vi "Current_Training_UI_3.10.22.vi"() -> ()   [LabVIEW 2021]
panel:
  out "Console out":string
  out "intro":picture
  out "view":picture
  out "training 2":picture
  out "sent string":string
  out "training":u16[](array[numeric])
  out "Motor Value":i32
  in  "Quit":bool
  out "Training String":string
  out "Tab Control":enum32{"Welcome", "View", "Train"}(tab)
  in  "Ready":bool
  out "Motor Position View":u8(knob) scale=0.0..4.0
  in  "TRAIN":bool
  out "Light Intensity % View":dbl(slide) scale=0.0..100.0
  out "?":u32(colorbox)
  in  "Done":bool
  in  "Motor Position":u8(knob) scale=0.0..4.0
  out "Light Intensity %":dbl(slide) scale=0.0..100.0
  in  "Training Data":bool
  in  "Upload":bool
  out "Light Intensity 2":u32(colorbox)
  out "table":picture
  in  "Done 2":bool
  out "concatenated string":string
  out "read buffer":string
  out "Motor":string
  out "Sensor":string
  out "Type":string
  out "Name":string
  out "read terminal buffer - view":string
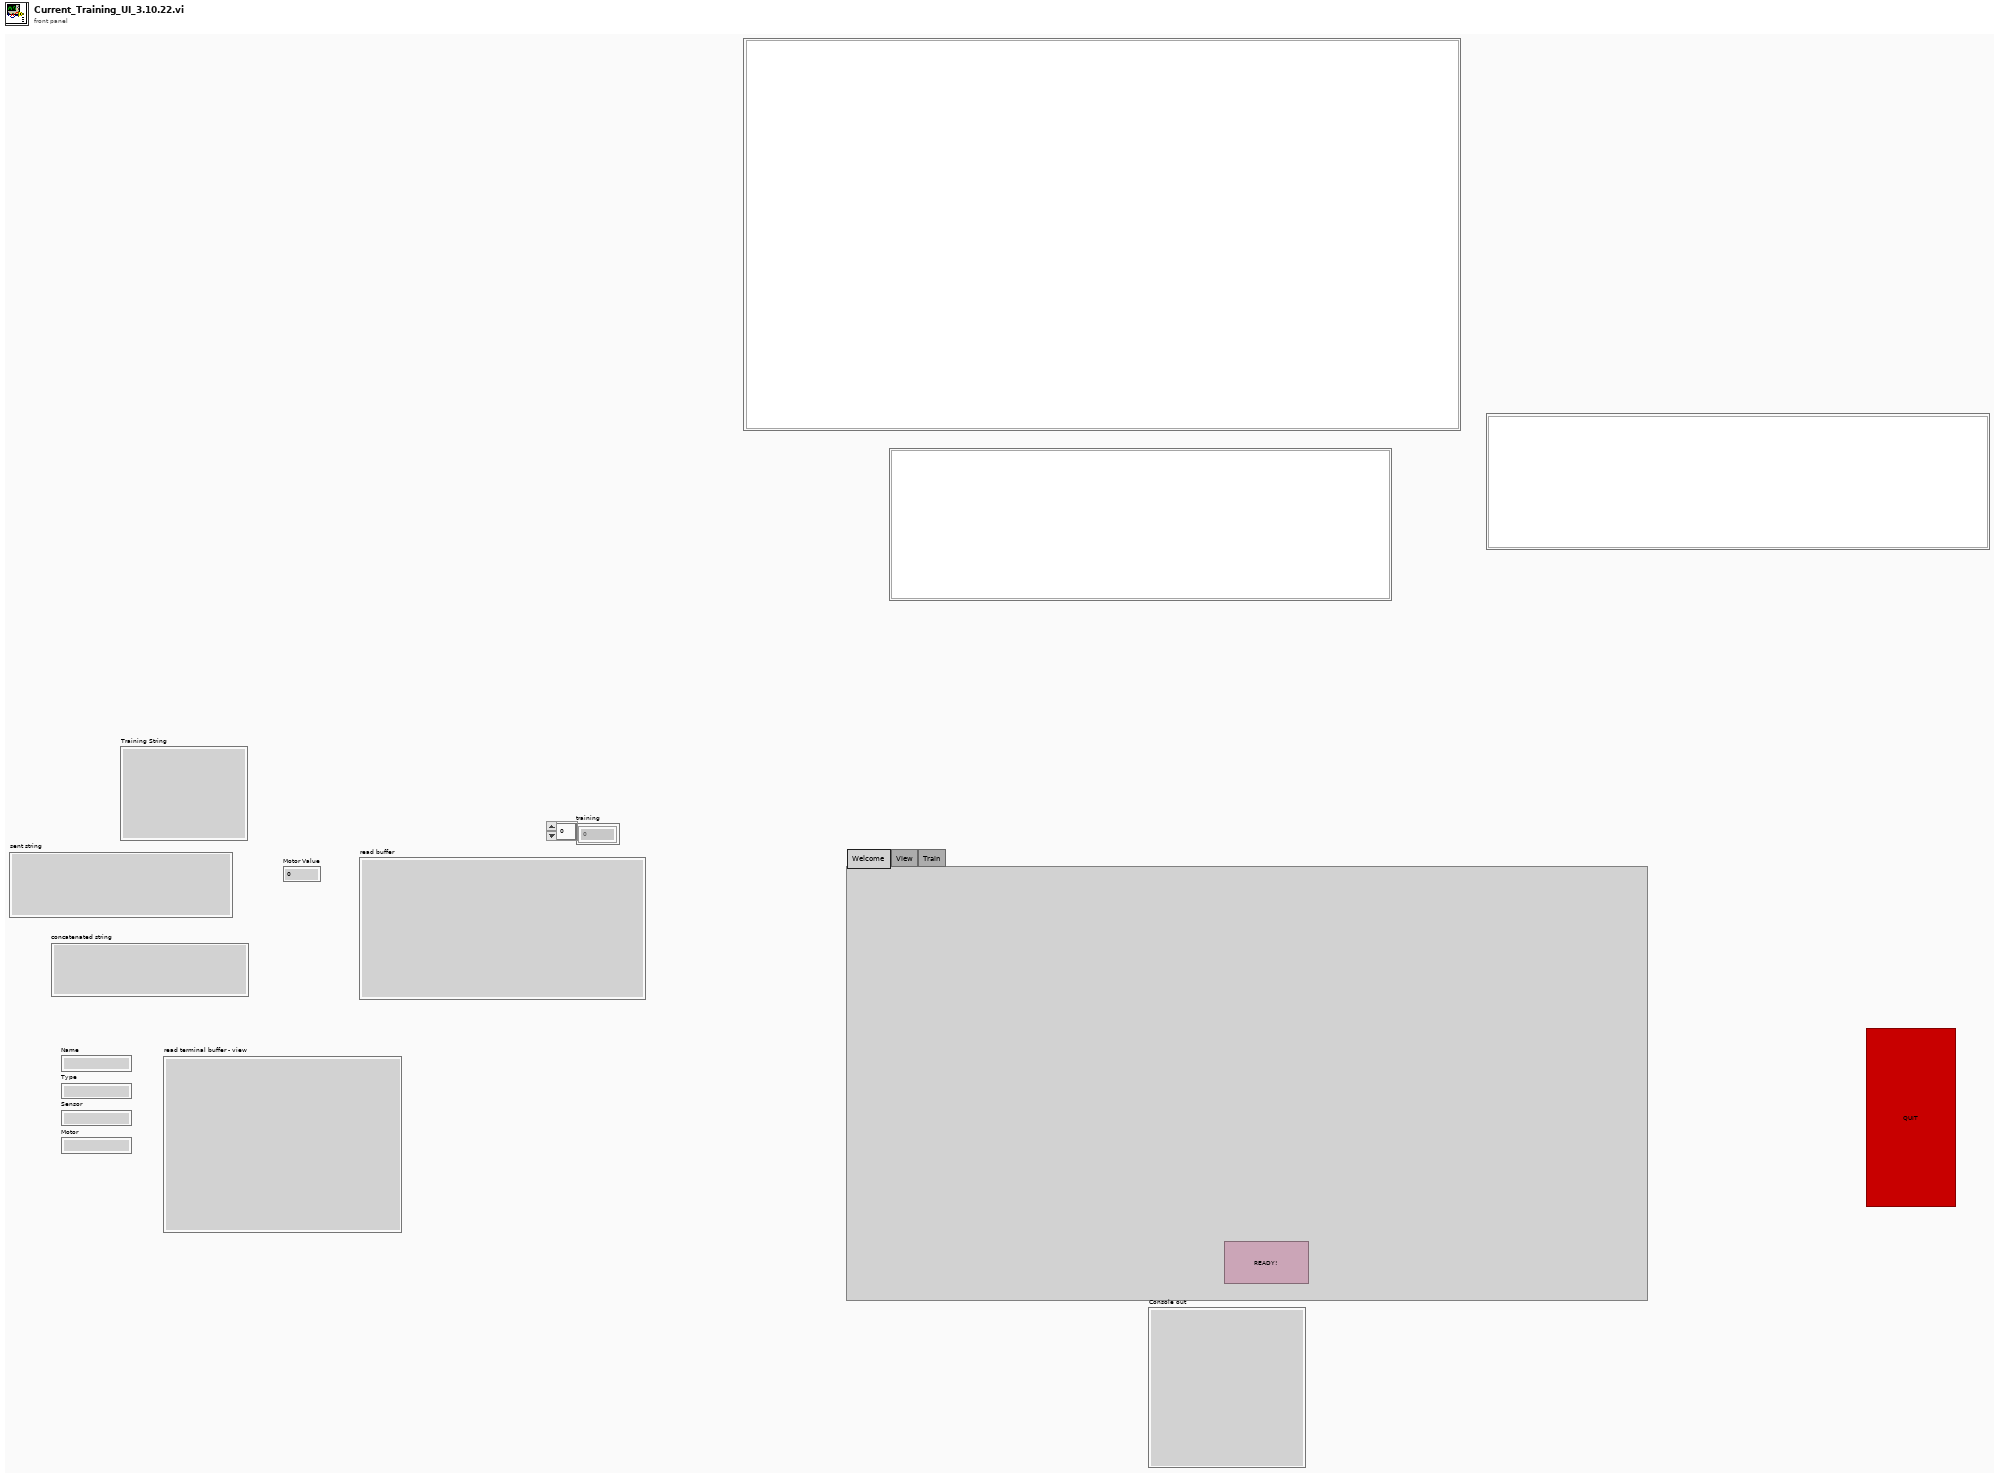
[diagram p1: front panel]
types:
  T1 = typedef "PythonCtrl.ctl" = cluster{"session":refnum<k35>, "PyPath":path, "Processor":enum16{"SPIKE", "Pi", "Pi_ssh"}}
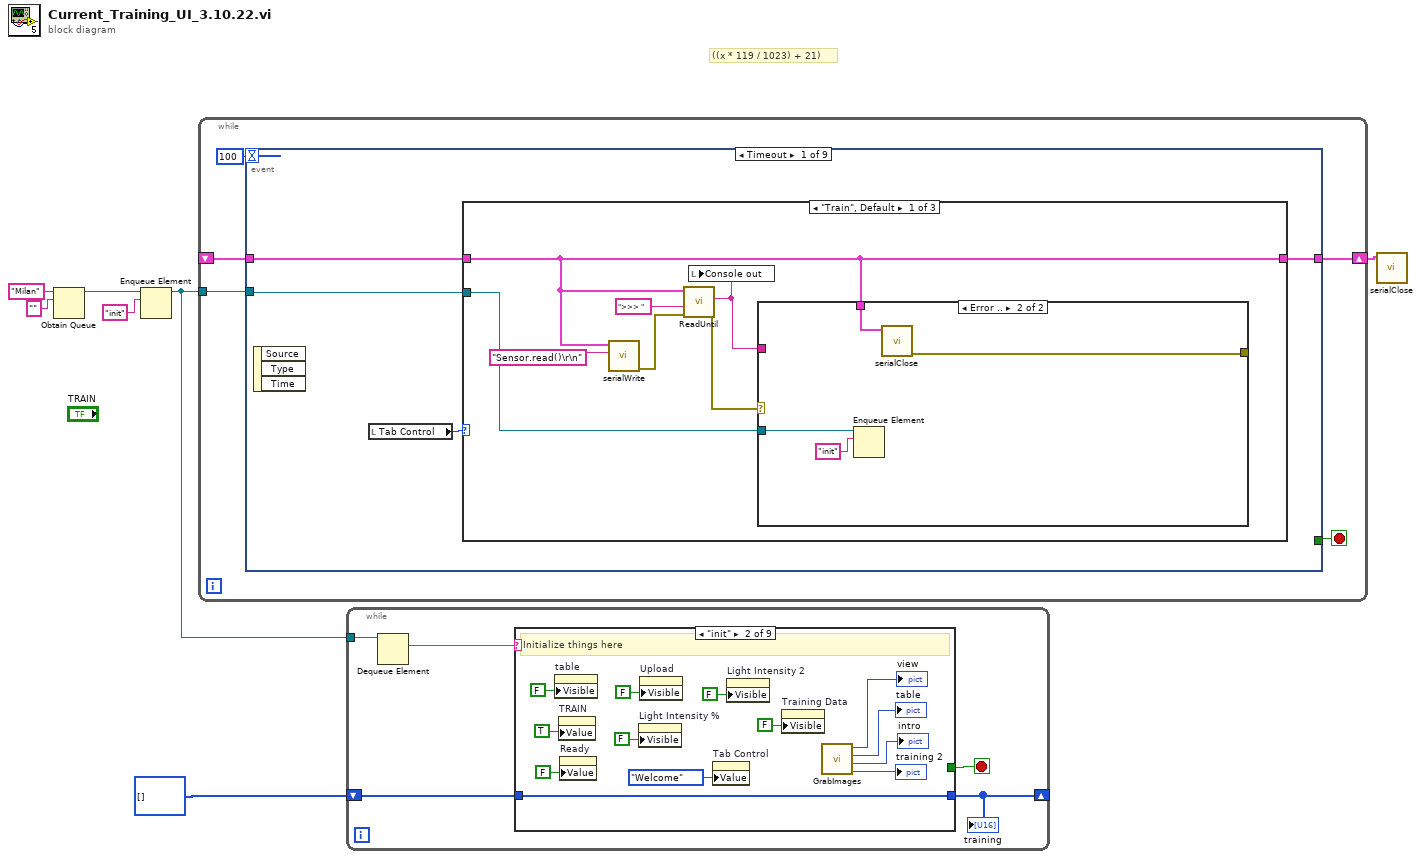
[diagram p0: block diagram]
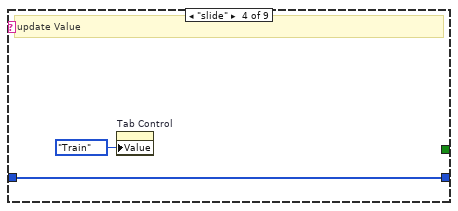
[diagram p4: hidden frame]
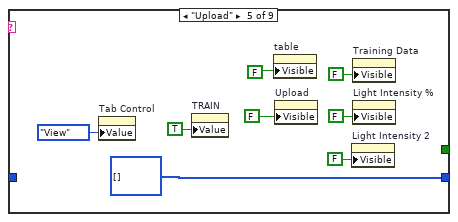
[diagram p5: hidden frame]
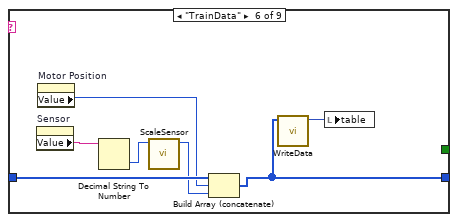
[diagram p6: hidden frame]
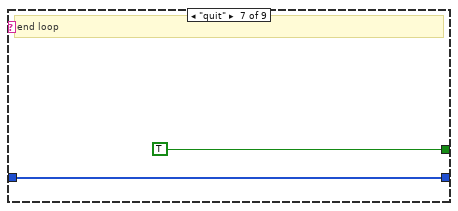
[diagram p7: hidden frame]
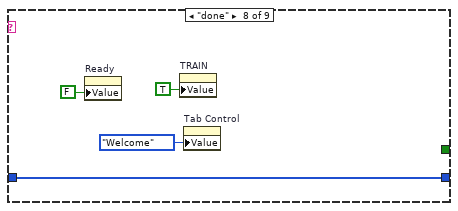
[diagram p8: hidden frame]
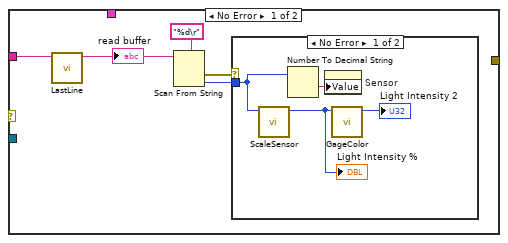
[diagram p10: hidden frame]
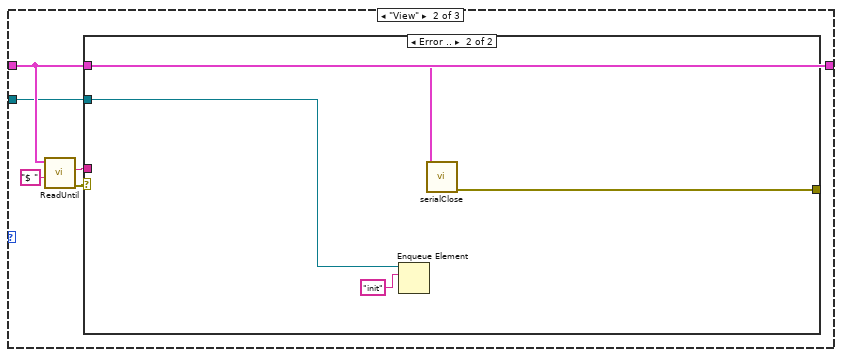
[diagram p12: hidden frame]
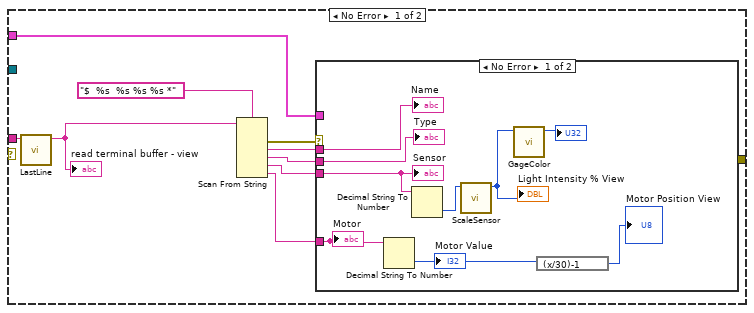
[diagram p13: hidden frame]
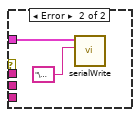
[diagram p14: hidden frame]
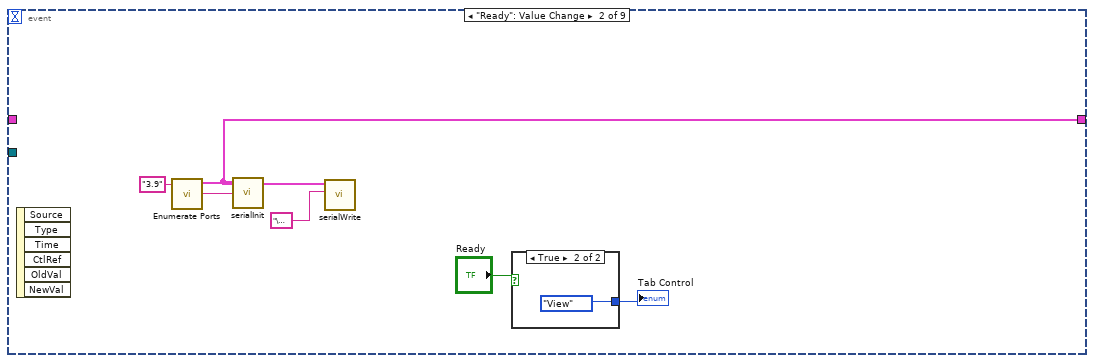
[diagram p16: hidden frame]
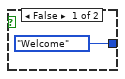
[diagram p17: hidden frame]
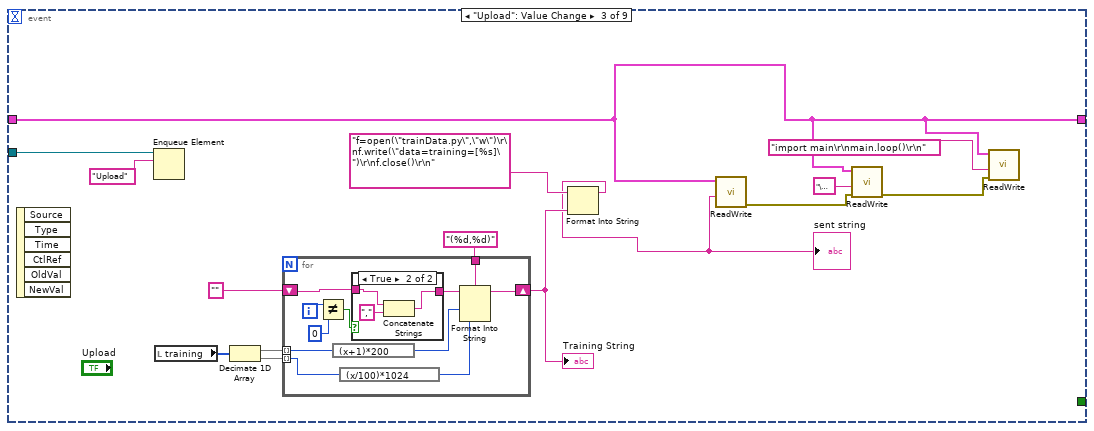
[diagram p18: hidden frame]
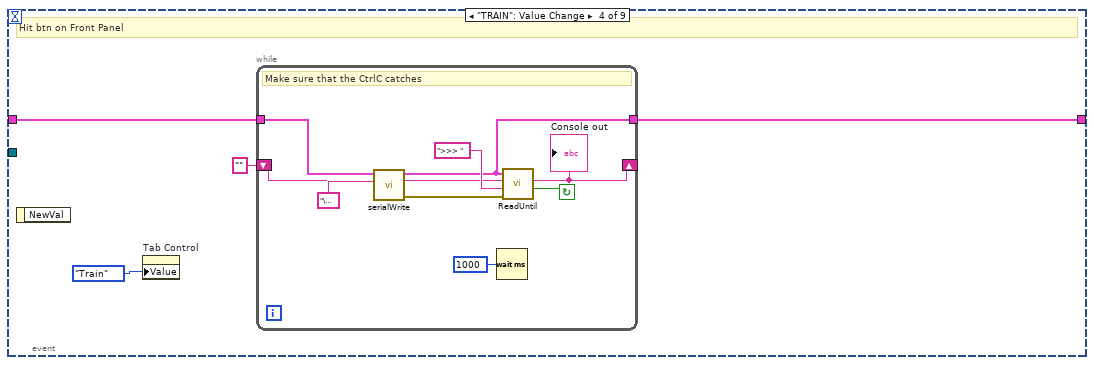
[diagram p20: hidden frame]
diagram:
  # "((x * 119 / 1023) + 21)"
  n1 = Obtain Queue(name (unnamed)="Milan", element data type="") -> (queue out=w7:refnum<queue>)  [unwired: 3 in, 2 out]
  n2 = Enqueue Element(queue=w7, element="init") -> (queue out=w3:refnum<queue>)  [unwired: 2 in, 2 out]
  n3 = while {
    tunnel: w3 -> [w12]
    shift-right: [w9] -> w2
    shift-left: _ -> [w10]
    stop <- w11 stop-if-true
    n4 = event shown="[0] Timeout" {
      selector: _ -> [_ _ _ _ _ _ _ _ _]
      dyn-events: _ -> [_ _ _ _ _ _ _ _ _]
      timeout: 100 -> [_ _ _ _ _ _ _ _ _]
      tunnel: w12 -> [w13 _ w89 _ w120 w130 w134 w138 w143]
      tunnel: [_ _ _ _ _ _ w133 TRUE ("Discard?") _] -> w11
      tunnel: w10 -> [w15 _ w75 w107 w119 w129 w132 w136 w140]
      tunnel: [w16 w67 w75 w106 w119 w129 w132 w136 w140] -> w9
      event Timeout {
        n5 = event-data() -> ()  [unwired: 1 in, 3 out]
        n6 = local read "Tab Control"() -> (w14:enum32{"Welcome", "View", "Train"})
        n7 = case shown="\"Train\", Default" w14 {
          tunnel: w15 -> [w18 w41 w66]
          tunnel: [w18 w41 w66] -> w16
          tunnel: w13 -> [w17 w37 _]
          frame "Train", Default {
            n8 = call "serialWrite.vi"("text"="Sensor.read()\r\n" ("write buffer"), "Python"=w18) -> ("error out"=w21:errorcluster)  [unwired: 8 in, 1 out]
            n9 = call "ReadUntil.vi"("error in (no error)"=w21, "EOL"=">>> ", "Python"=w18) -> ("error out"=w19:errorcluster, "Console out"=w20:string)  [unwired: 6 in, 1 out]
            n10 = local write "Console out"(w20) -> ()
            n11 = case shown="Error .." w19 {
              tunnel: w20 -> [w24 _]
              tunnel: w18 -> [_ w35]
              tunnel: w17 -> [_ w34]
              tunnel: [_ w33] -> _
              frame No Error {
                n12 = call "LastLine.vi"("Reply"=w24) -> ("String"=w25:string)  [unwired: 10 in]
                "read buffer" <- w25
                n13 = Scan From String(format string="%d\r", input string=w25) -> (error out=w28:errorcluster, output 1=w27:i32)  [unwired: 3 in, 2 out]
                n14 = case shown="No Error" w28 {
                  tunnel: w27 -> [w30 _]
                  frame No Error {
                    n15 = call "ScaleSensor.vi"("value"=w30) -> ("scaled value"=w29:u16)  [unwired: 10 in]
                    "Light Intensity %" <- w29
                    n16 = Number To Decimal String(number=w30) -> (decimal integer string=w32:string)  [unwired: 1 in]
                    n17 = property on="Sensor" class="Str"("Value"=w32) -> ()  [unwired: 2 in, 2 out]
                    n18 = call "GageColor.vi"("value"=w29) -> ("Color Box"=→"Light Intensity 2":u32)  [unwired: 10 in]
                  }
                  frame Error {
                  }
                }
              }
              frame Error {
                n19 = Enqueue Element(queue=w34, element="init") -> ()  [unwired: 2 in, 3 out]
                n20 = call "serialClose.vi"("Python in"=w35) -> ("error out"=w33:errorcluster)  [unwired: 10 in]
              }
            }
          }
          frame "View" {
            n21 = call "ReadUntil.vi"("EOL"="$ ", "Python"=w41) -> ("error out"=w39:errorcluster, "Console out"=w40:string)  [unwired: 7 in, 1 out]
            n22 = case shown="Error .." w39 {
              tunnel: w40 -> [w44 _]
              tunnel: w41 -> [w42 w64]
              tunnel: w37 -> [_ w63]
              tunnel: [_ w62] -> _
              frame No Error {
                n23 = call "LastLine.vi"("Reply"=w44) -> ("String"=w43:string)  [unwired: 10 in]
                "read terminal buffer - view" <- w43
                n24 = Scan From String(format string="$  %s  %s %s %s *", input string=w43) -> (error out=w50:errorcluster, output 1=w46:string, output 2=w47:string, output 3=w48:string, output 4=w49:string)  [unwired: 6 in, 2 out]
                n25 = case shown="No Error" w50 {
                  tunnel: w46 -> [w59 _]
                  tunnel: w47 -> [w58 _]
                  tunnel: w48 -> [w57 _]
                  tunnel: w49 -> [w54 _]
                  tunnel: w42 -> [_ w61]
                  frame No Error {
                    n26 = Decimal String To Number(string=w54) -> (number=w52:i32)  [unwired: 2 in, 1 out]
                    "Motor Value" <- w52
                    n27 = Decimal String To Number(string=w57) -> (number=w56:i32)  [unwired: 2 in, 1 out]
                    n28 = call "ScaleSensor.vi"("value"=w56) -> ("scaled value"=w53:u16)  [unwired: 10 in]
                    "Light Intensity % View" <- w53
                    n29 = call "GageColor.vi"("value"=w53) -> ("Color Box"=→"?":u32)  [unwired: 10 in]
                    n30 = expression code="(x/30)-1"(w52) -> (→"Motor Position View":i32)
                    "Name" <- w59
                    "Type" <- w58
                    "Sensor" <- w57
                    "Motor" <- w54
                  }
                  frame Error {
                    n31 = call "serialWrite.vi"("text"="\u0003", "Python"=w61) -> ()  [unwired: 8 in, 2 out]
                  }
                }
              }
              frame Error {
                n32 = Enqueue Element(queue=w63, element="init") -> ()  [unwired: 2 in, 3 out]
                n33 = call "serialClose.vi"("Python in"=w64) -> ("error out"=w62:errorcluster)  [unwired: 10 in]
              }
            }
          }
          frame "Welcome" {
          }
        }
      }
      event "Ready": Value Change {
        n34 = event-data() -> ()  [unwired: 1 in, 6 out]
        n35 = call "Enumerate Ports.vi"("Python version"="3.9") -> ("guess"=w70:string, "Python"=w67:T1)  [unwired: 6 in, 3 out]
        n36 = call "serialInit.vi"("Port"=w70, "Python"=w67) -> ()  [unwired: 8 in, 2 out]
        n37 = call "serialWrite.vi"("text"="\u0004" ("write buffer"), "Python"=w67) -> ()  [unwired: 8 in, 2 out]
        n38 = case shown="True" "Ready" {
          tunnel: [enum32{"Welcome", "View", "Train"}."Welcome" ("Tab Control") enum32{"Welcome", "View", "Train"}."View" ("Tab Control")] -> w71
          frame False {
          }
          frame True {
          }
        }
        "Tab Control" <- w71
      }
      event "Upload": Value Change {
        n39 = event-data() -> ()  [unwired: 1 in, 6 out]
        n40 = Enqueue Element(queue=w89, element="Upload") -> ()  [unwired: 2 in, 3 out]
        n41 = local read "training"() -> (w87:u16[])
        n42 = Decimate 1D Array(w87) -> (w85:u16[], w84:u16[])
        n43 = for {
          tunnel: "(%d,%d)" ("format string") -> [w100]
          tunnel: w85 -> [w93] mode=indexing
          tunnel: w84 -> [w91] mode=indexing
          shift-right: [w99] -> w82
          shift-left: "" -> [w98]
          i -> [w95]
          n44 = Not Equal?(x=w95, y=0) -> (x != y?=w96:bool)
          n45 = expression code="(x+1)*200"(w93) -> (w92:u16)
          n46 = expression code="(x/100)*1024"(w91) -> (w90:u16)
          n47 = case shown="True" w96 {
            tunnel: w98 -> [w101 w103]
            tunnel: [w101 w102] -> w97
            frame False {
            }
            frame True {
              n48 = Concatenate Strings(w103, "," ("string")) -> (w102:string)
            }
          }
          n49 = Format Into String(format string=w100, initial string=w97, w92, w90) -> (resulting string=w99:string)  [unwired: 1 in, 1 out]
        }
        "Training String" <- w82
        n50 = Format Into String(format string="f=open(\"trainData.py\",\"w\")\r\nf.write(\"data=training=[%s]\")\r\nf.close()\r\n" ("string"), w82) -> (resulting string=w80:string)  [unwired: 2 in, 1 out]
        "sent string" <- w80
        n51 = call "ReadWrite.vi"("Code"=w80, "Python"=w75) -> ("error out"=w76:errorcluster)  [unwired: 8 in, 1 out]
        n52 = call "ReadWrite.vi"("error in (no error)"=w76, "Code"="\u0004" ("text"), "Python"=w75) -> ("error out"=w77:errorcluster)  [unwired: 7 in, 1 out]
        n53 = call "ReadWrite.vi"("error in (no error)"=w77, "Code"="import main\r\nmain.loop()\r\n" ("text"), "Python"=w75) -> ()  [unwired: 7 in, 2 out]
      }
      event "TRAIN": Value Change {
        # "Hit btn on Front Panel"
        n54 = event-data() -> ()  [unwired: 1 in, 1 out]
        n55 = property on="Tab Control" class="TabCtl (strict)"("Value"=enum32{"Welcome", "View", "Train"}."Train" ("Tab Control")) -> ()  [unwired: 2 in, 2 out]
        n56 = while {
          tunnel: w107 -> [w111]
          tunnel: [w111] -> w106
          shift-right: [w110] -> _
          shift-left: "" ("Console out") -> [w109]
          stop <- w113 continue-if-true
          # "Make sure that the CtrlC catches"
          n57 = call "serialWrite.vi"("text"="\u0003" ("write buffer"), "Python"=w111) -> ("error out"=w114:errorcluster)  [unwired: 8 in, 1 out]
          n58 = Wait (ms)(milliseconds to wait=u32 1000) -> ()  [unwired: 1 out]
          n59 = call "ReadUntil.vi"("error in (no error)"=w114, "EOL"=">>> ", "Console in"=w109, "Python"=w111) -> ("timed out?"=w113:bool, "Console out"=w110:string)  [unwired: 5 in, 1 out]
          "Console out" <- w110
        }
      }
      event "Training Data": Value Change {
        n60 = event-data() -> ()  [unwired: 1 in, 6 out]
        n61 = Enqueue Element(queue=w120, element="TrainData") -> ()  [unwired: 2 in, 3 out]
        n62 = property on="table" class="Pict"("Visible"=TRUE) -> ()  [unwired: 2 in, 2 out]
        n63 = property on="Upload" class="Bool (strict)"("Visible"=TRUE) -> ()  [unwired: 2 in, 2 out]
      }
      event "Motor Position": Value Change {
        # "Slide slid on Front Panel"
        n64 = event-data() -> ()  [unwired: 1 in, 6 out]
        n65 = Enqueue Element(queue=w130, element="slide") -> ()  [unwired: 2 in, 3 out]
        n66 = property on="Training Data" class="Bool"("Visible"=TRUE) -> ()  [unwired: 2 in, 2 out]
        n67 = expression code="(x+1)*30"("Motor Position") -> (w125:u8)
        n68 = Format Into String(format string="pwm2.duty(%d)\r\n", w125) -> (resulting string=w127:string)  [unwired: 2 in, 1 out]
        "concatenated string" <- w127
        n69 = property on="Light Intensity %" class="Slide (strict)"("Visible"=TRUE) -> ()  [unwired: 2 in, 2 out]
        n70 = call "serialWrite.vi"("text"=w127, "Python"=w129) -> ()  [unwired: 8 in, 2 out]
        n71 = property on="Light Intensity 2" class="ColBox"("Visible"=TRUE) -> ()  [unwired: 2 in, 2 out]
      }
      event Panel Close? {
        w133 = TRUE ("Discard?")
        # "Closed the Window"
        n72 = event-data() -> ()  [unwired: 1 in, 2 out]
        n73 = Enqueue Element(queue=w134, element="done") -> ()  [unwired: 2 in, 3 out]
        n74 = event-data("Discard?"=w133) -> ()  [unwired: 1 in, 1 out]
      }
      event "Quit": Value Change {
        # "hit Done btn"
        n75 = event-data() -> ()  [unwired: 1 in, 2 out]
        n76 = Enqueue Element(queue=w138, element="quit") -> ()  [unwired: 2 in, 3 out]
      }
      event "Done", "Done 2": Value Change {
        n77 = event-data() -> ()  [unwired: 1 in, 6 out]
        n78 = Enqueue Element(queue=w143, element="done") -> ()  [unwired: 2 in, 3 out]
        n79 = call "ReadWrite.vi"("Code"="\u0004" ("text"), "Python"=w140) -> ()  [unwired: 8 in, 2 out]
        n80 = call "ReadWrite.vi"("Code"="import main\r\nmain.loop()\r\n" ("text"), "Python"=w140) -> ()  [unwired: 8 in, 2 out]
      }
    }
  }
  n81 = while {
    tunnel: w3 -> [w149]
    shift-right: [w145] -> _
    shift-left: u16[] [] ("initialized array") -> [w146]
    stop <- w147 stop-if-true
    n82 = Dequeue Element(queue=w149) -> (element=w148:string)  [unwired: 2 in, 3 out]
    n83 = case shown="\"init\"" w148 {
      tunnel: [_ _ _ _ _ _ TRUE ("Discard?") _ _] -> w147
      tunnel: w146 -> [w150 w163 w164 w166 _ w181 w182 w186 w188]
      tunnel: [w150 w163 w164 w166 u16[] [] ("initialized array") w177 w182 w186 w188] -> w145
      frame Default {
      }
      frame "init" {
        # "Initialize things here"
        n84 = property on="table" class="Pict"("Visible"=FALSE) -> ()  [unwired: 2 in, 2 out]
        n85 = property on="TRAIN" class="Bool (strict)"("Value"=TRUE ("Train")) -> ()  [unwired: 2 in, 2 out]
        n86 = property on="Ready" class="Bool (strict)"("Value"=FALSE ("Ready")) -> ()  [unwired: 2 in, 2 out]
        n87 = property on="Light Intensity %" class="Slide (strict)"("Visible"=FALSE) -> ()  [unwired: 2 in, 2 out]
        n88 = property on="Upload" class="Bool (strict)"("Visible"=FALSE) -> ()  [unwired: 2 in, 2 out]
        n89 = property on="Tab Control" class="TabCtl (strict)"("Value"=enum32{"Welcome", "View", "Train"}."Welcome" ("Tab Control")) -> ()  [unwired: 2 in, 2 out]
        n90 = property on="Light Intensity 2" class="ColBox"("Visible"=FALSE) -> ()  [unwired: 2 in, 2 out]
        n91 = property on="Training Data" class="Bool"("Visible"=FALSE) -> ()  [unwired: 2 in, 2 out]
        n92 = call "GrabImages.vi"() -> ("Training Instructions"=→"training 2":picture, "Intro"=→"intro":picture, "Table"=→"table":picture, "View Instructions"=→"view":picture)  [unwired: 8 in]
      }
      frame "Train" {
        # "reset LED"
      }
      frame "slide" {
        # "update Value"
        n93 = property on="Tab Control" class="TabCtl (strict)"("Value"=enum32{"Welcome", "View", "Train"}."Train" ("Tab Control")) -> ()  [unwired: 2 in, 2 out]
      }
      frame "Upload" {
        n94 = property on="Tab Control" class="TabCtl (strict)"("Value"=enum32{"Welcome", "View", "Train"}."View" ("Tab Control")) -> ()  [unwired: 2 in, 2 out]
        n95 = property on="TRAIN" class="Bool (strict)"("Value"=TRUE ("TRAIN")) -> ()  [unwired: 2 in, 2 out]
        n96 = property on="table" class="Pict"("Visible"=FALSE) -> ()  [unwired: 2 in, 2 out]
        n97 = property on="Upload" class="Bool (strict)"("Visible"=FALSE) -> ()  [unwired: 2 in, 2 out]
        n98 = property on="Light Intensity 2" class="ColBox"("Visible"=FALSE) -> ()  [unwired: 2 in, 2 out]
        n99 = property on="Training Data" class="Bool"("Visible"=FALSE) -> ()  [unwired: 2 in, 2 out]
        n100 = property on="Light Intensity %" class="Slide (strict)"("Visible"=FALSE) -> ()  [unwired: 2 in, 2 out]
      }
      frame "TrainData" {
        n101 = property on="Sensor" class="Str"() -> ("Value"=w180:string)  [unwired: 2 in, 2 out]
        n102 = property on="Motor Position" class="Knob (strict)"() -> ("Value"=w175:u8)  [unwired: 2 in, 2 out]
        n103 = Decimal String To Number(string=w180) -> (number=w179:i32)  [unwired: 2 in, 1 out]
        n104 = call "ScaleSensor.vi"("value"=w179) -> ("scaled value"=w178:u16)  [unwired: 10 in]
        n105 = Build Array (concatenate)(w181, w175, w178) -> (w177:u16[])
        n106 = call "WriteData.vi"("Array"=w177) -> ("Table"=w176:picture)  [unwired: 10 in]
        n107 = local write "table"(w176) -> ()
      }
      frame "quit" {
        # "end loop"
      }
      frame "done" {
        n108 = property on="Ready" class="Bool (strict)"("Value"=FALSE ("Ready")) -> ()  [unwired: 2 in, 2 out]
        n109 = property on="TRAIN" class="Bool (strict)"("Value"=TRUE ("TRAIN")) -> ()  [unwired: 2 in, 2 out]
        n110 = property on="Tab Control" class="TabCtl (strict)"("Value"=enum32{"Welcome", "View", "Train"}."Welcome" ("Tab Control")) -> ()  [unwired: 2 in, 2 out]
      }
      frame "" {
      }
    }
    "training" <- w145
  }
  n111 = call "serialClose.vi"("Python in"=w2) -> ()  [unwired: 10 in, 1 out]
